vi "DWF MSO Query Analog Edge Trigger.vi"(0 "Instrument Handle In":u32, 11 "Error In":errorcluster caption="Error In (no error)", 12 "Trigger Instance":i32(ring) caption="Trigger Instance (A)" items=["A", "B"]) -> (3 "Trigger Hysteresis":dbl, 4 "Instrument Handle Out":u32, 6 "Trigger Source":string caption="Trigger Pattern", 8 "Trigger Slope":i32(ring) items=["Rising", "Falling", "Either"], 10 "Trigger Level":dbl, 15 "Error Out":errorcluster)   [LabVIEW 2015, in "DigilentWF.lvlib"]
doc: "Indicates the analog edge trigger configuration of the specified instance."
uses:
  <vilib>/DigilentWF/DigilentWF.lvlib
  dwf.dll
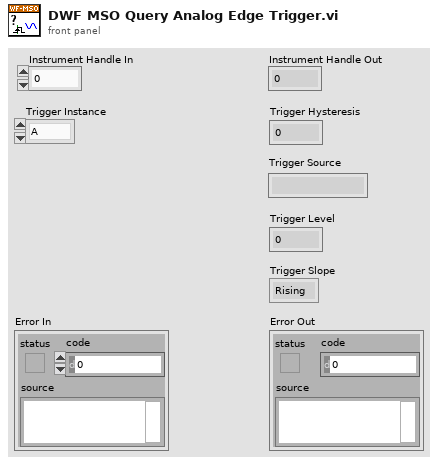
[diagram p1: front panel]
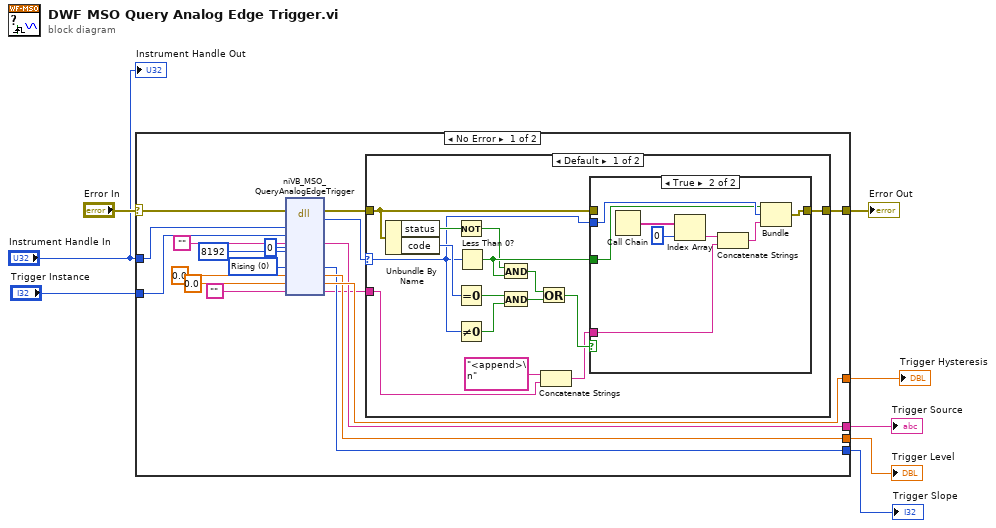
[diagram p0: block diagram]
diagram:
  n1 = case "outter_case" shown="No Error" "Error In" {
    selector: "Error In" -> [w26 w52]
    tunnel: [w23 w52] -> w7
    tunnel: "Instrument Handle In" -> [w12 _]
    tunnel: "Trigger Instance" -> [w22 _]
    tunnel: [w18 _] -> w4
    tunnel: [w17 _] -> w1
    tunnel: [w16 _] -> w3
    tunnel: [w15 _] -> w2
    frame No Error {
      w19 = 0 items=["Rising", "Falling", "Either"] ("Trigger Slope")
      n2 = dll-call lib="dwf.*" fn="niVB_MSO_QueryAnalogEdgeTrigger"(error in=w26, "InstrumentHandle"=w12, "TriggerInstance"=w22, "TriggerSource"="", "cTriggerSource"=8192, "pTriggerSource"=0, "TriggerSlope"=w19, "TriggerLevel"=0.0 ("Trigger Level"), "TriggerHysteresis"=0.0 ("Trigger Hysteresis"), "szError"="") -> (error out=w25:errorcluster, "return type"=w24:i32, "TriggerSource"=w17:string, "TriggerSlope"=w15:i32, "TriggerLevel"=w16:dbl, "TriggerHysteresis"=w18:dbl, "szError"=w13:string)  [unwired: 6 in, 1 out]
      n3 = case "inner_case" shown="Default" w24 {
        selector: w24 -> [w31 _]
        tunnel: w25 -> [w32 w51]
        tunnel: [w28 w51] -> w23
        tunnel: w13 -> [w27 _]
        frame Default {
          n4 = Unbundle By Name(w32) -> ("status"=w36:bool, "code"=w40:i32)
          n5 = Not(x=w36) -> (.not. x?=w39:bool)
          n6 = Equal To 0?(x=w40) -> (x = 0?=w35:bool)
          n7 = Not Equal To 0?(x=w31) -> (x != 0?=w38:bool)
          n8 = Less Than 0?(x=w31) -> (x < 0?=w41:bool)
          n9 = And(x=w39, y=w41) -> (x .and. y?=w37:bool)
          n10 = And(x=w35, y=w38) -> (x .and. y?=w34:bool)
          n11 = Or(x=w37, y=w34) -> (x .or. y?=w33:bool)
          n12 = Concatenate Strings("<append>\n" ("string"), w27) -> (w30:string)
          n13 = case shown="True" w33 {
            tunnel: [w42 w49] -> w28
            tunnel: w31 -> [_ w48]
            tunnel: w41 -> [_ w47]
            tunnel: w32 -> [w42 _]
            tunnel: w30 -> [_ w43]
            frame False {
            }
            frame True {
              n14 = Call Chain() -> (call chain=w46:string[])
              n15 = Index Array(array=w46, index=0) -> (element=w45:string)
              n16 = Concatenate Strings(w45, w43) -> (w50:string)
              n17 = Bundle(w47, "return type"=w48, w50) -> (w49:cluster{bool, "return type":i32, string})  [unwired: 1 out]
            }
          }
        }
        frame 0 {
        }
      }
    }
    frame Error {
    }
  }
  "Error Out" <- w7
  "Trigger Hysteresis" <- w4
  "Trigger Level" <- w3
  "Trigger Slope" <- w2
  "Trigger Source" <- w1
  "Instrument Handle Out" <- "Instrument Handle In"
